vi "SMBus Read Byte.vi"(6 "PEC":u8, 7 "SlaveAddr":u8, 9 "SMBUSIndex":i32, 10 "DevIndex":i32, 11 "DevType":i32) -> (2 "function return":i32, 3 "pData":u8)   [LabVIEW 2010, in "ControlSMBus.lvlib"]
doc: "int WINAPI SMBus_ReadByte(int DevType,int DevIndex,int SMBUSIndex,unsigned char SlaveAddr,unsigned char *pData,unsigned char PEC);"
uses:
  ControlSMBus.lvlib
  ControlSMBus/Ginkgo_Driver.dll
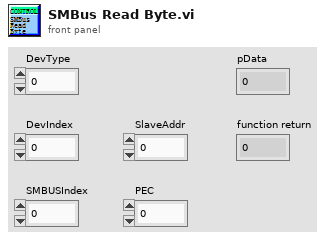
[diagram p1: front panel]
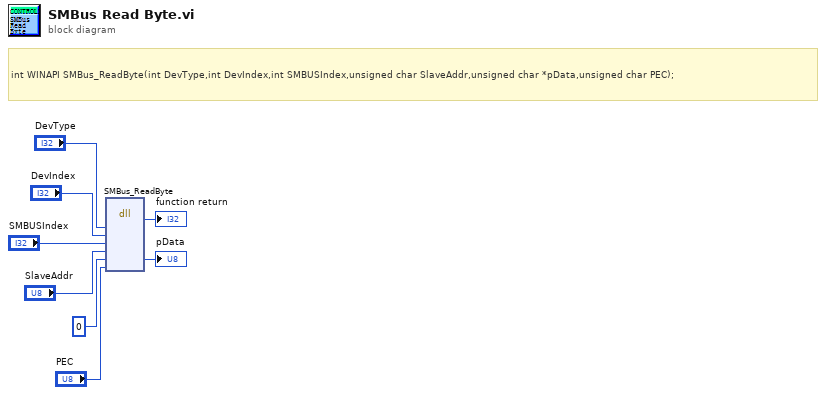
[diagram p0: block diagram]
diagram:
  # "int WINAPI SMBus_ReadByte(int DevType,int DevIndex,int SMBUSIndex,unsigned char SlaveAddr,unsigned char *pData,unsigned char PEC);"
  n1 = dll-call lib="E:/Project/vt_ginkgo/truck/Ginkgo Driver/vs2010/Ginkgo_USB-I2C&SPI&CAN_API_v2.0.3.3/lib/labview_32bit/ControlSMBus/Ginkgo_Driver.*" fn="SMBus_ReadByte"("DevType"="DevType", "DevIndex"="DevIndex", "SMBUSIndex"="SMBUSIndex", "SlaveAddr"="SlaveAddr", "pData"=u8 0, "PEC"="PEC") -> (→"function return":i32, "pData"=→"pData":u8)  [unwired: 8 in, 2 out]
